vi "Parse DAT String.vi"(8 "error in (no error)":errorcluster, 10 "header length":i32=11, 11 "spreadsheet string":string[][](array[string])) -> (0 "error out":errorcluster, 2 "Notes":string, 3 "Data (Dictionary)":T1[](array[typedef]))   [LabVIEW 2019, in "Data.DAT.lvclass"]
uses:
  Data.DAT.lvclass
  Data/Typedefs/Dictionary--cluster.ctl
  Data/Data.lvclass
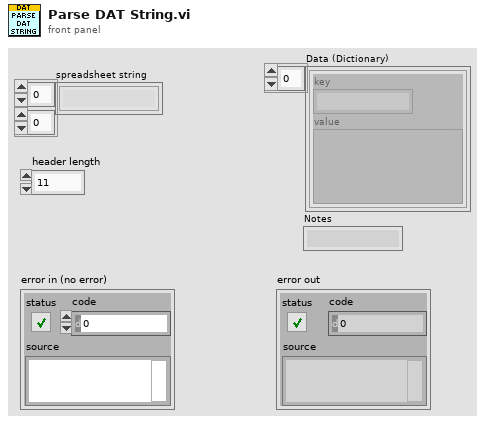
[diagram p1: front panel]
types:
  T1 = typedef "Data.lvclass/Dictionary--cluster.ctl" = cluster{"key":string, "value":variant}
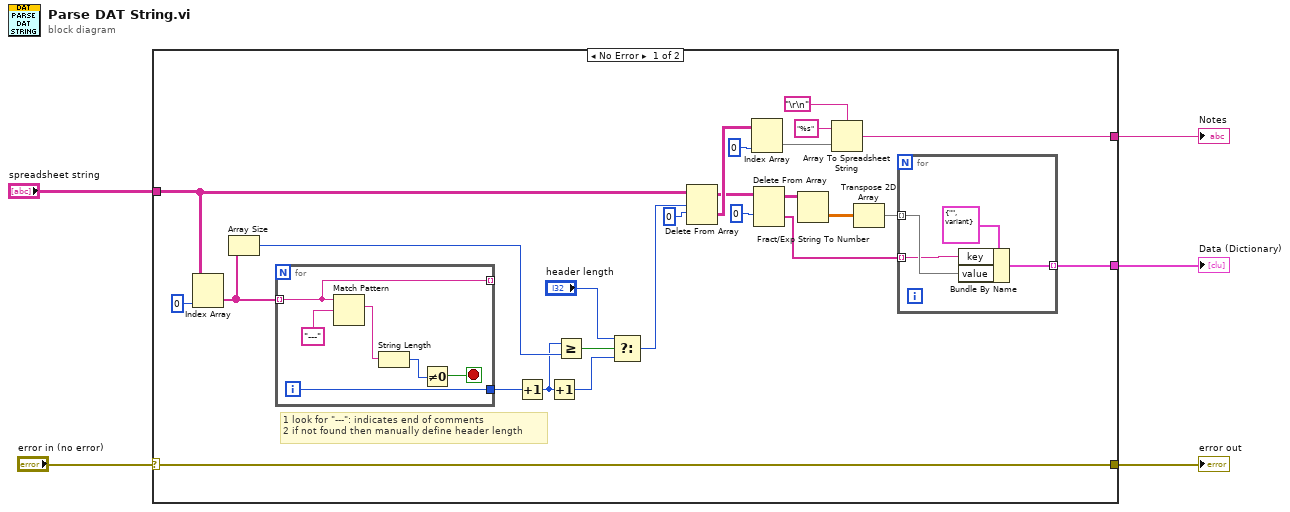
[diagram p0: block diagram]
diagram:
  n1 = case shown="No Error" "error in (no error)" {
    selector: "error in (no error)" -> [w6 w41]
    tunnel: [w30 _] -> w5
    tunnel: [w29 _] -> w4
    tunnel: "spreadsheet string" -> [w7 _]
    tunnel: [w6 w41] -> w1
    frame No Error {
      # "1 look for \"---\": indicates end of comments\n2 if not found then manually define header length"
      n2 = Index Array(array=w7, index (col)=0 ("disabled index (col)")) -> (element=w19:string[])  [unwired: 1 in]
      n3 = Array Size(array=w19) -> (size(s)=w22:i32)
      n4 = for {
        tunnel: w19 -> [w31] mode=indexing
        tunnel: [w32] -> w18
        tunnel: [w31] -> _ mode=indexing
        i -> [w32]
        stop <- w34 stop-if-true
        n5 = Match Pattern(string=w31, regular expression="---") -> (match substring=w35:string)  [unwired: 4 out]
        n6 = String Length(string=w35) -> (length=w33:i32)
        n7 = Not Equal To 0?(x=w33) -> (x != 0?=w34:bool)
      }
      n8 = Increment(x=w18) -> (x+1=w20:i32)
      n9 = Increment(x=w20) -> (x+1=w23:i32)
      n10 = Greater Or Equal?(x=w20, y=w22) -> (x >= y?=w21:bool)
      n11 = Select(t="header length", s=w21, f=w23) -> (s? t:f=w25:i32)
      n12 = Delete From Array(array=w7, length=w25, index (row)=0) -> (deleted portion=w15:string[][], array with subset deleted=w11:string[][])  [unwired: 1 in]
      n13 = Index Array(array=w15, index (col)=0 ("disabled index (col)")) -> (element=w16:string[])  [unwired: 1 in]
      n14 = Delete From Array(array=w11, index (row)=0) -> (deleted portion=w26:string[], array with subset deleted=w10:string[][])  [unwired: 2 in]
      n15 = Fract/Exp String To Number(string=w10) -> (number=w27:dbl[][])  [unwired: 3 in, 1 out]
      n16 = Array To Spreadsheet String(delimiter (Tab)="\r\n", array=w16, 3:"%s" ("format string")) -> (spreadsheet string=w30:string)
      n17 = Transpose 2D Array(2D array=w27) -> (transposed array=w28:dbl[][])
      n18 = for {
        tunnel: w26 -> [w37] mode=indexing
        tunnel: w28 -> [w38] mode=indexing
        tunnel: [w40] -> w29 mode=indexing
        n19 = Bundle By Name(cluster=T1 {"key"="", "value"=variant} ("key-value"), "key"=w37, "value"=w38) -> (w40:T1)
      }
    }
    frame Error {
    }
  }
  "Notes" <- w5
  "Data (Dictionary)" <- w4
  "error out" <- w1
